vi "Tree_Get All Child Tags.vi"(8 "error in (no error)":errorcluster, 10 "Parent Tag":string, 11 "Tree Refnum":refnum<vi>) -> (0 "error out":errorcluster, 2 "All Child Tags":string[](array[string]), 3 "dup Tree Refnum":refnum<vi>)   [LabVIEW 2017]
doc: "This VI takes a tree reference and a parent tag value, and returns a string array with the tags of all children (including sub-children) of the given parent tag."
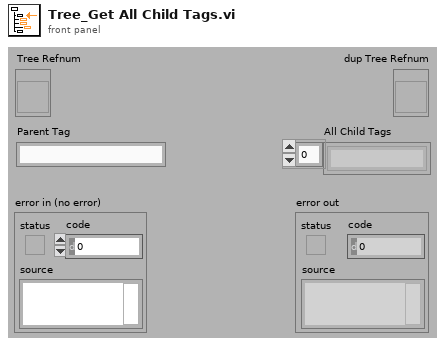
[diagram p1: front panel]
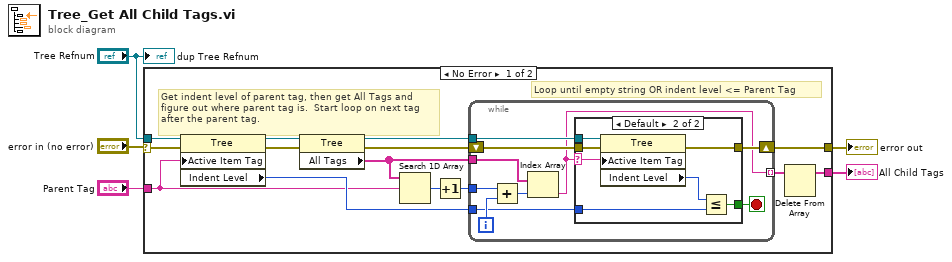
[diagram p0: block diagram]
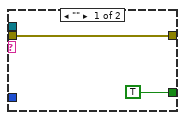
[diagram p2: hidden frame]
diagram:
  n1 = case shown="No Error" "error in (no error)" {
    selector: "error in (no error)" -> [w18 w39]
    tunnel: [w9 w39] -> w4
    tunnel: "Tree Refnum" -> [w19 _]
    tunnel: "Parent Tag" -> [w6 _]
    tunnel: [w11 _] -> w1
    frame No Error {
      # "Loop until empty string OR indent level <= Parent Tag"
      # "Get indent level of parent tag, then get All Tags and\nfigure out where parent tag is.  Start loop on next tag\nafter the parent tag."
      n2 = property class="Tree"(reference=w19, error in=w18, "Active Item Tag"=w6) -> (reference out=w16:refnum<vi>, error out=w17:errorcluster, "Indent Level"=w7:i32)
      n3 = property class="Tree"(reference=w16, error in=w17) -> (reference out=w8:refnum<vi>, error out=w10:errorcluster, "All Tags"=w14:string[])
      n4 = Search 1D Array(1D array=w14, element=w6) -> (index of element=w15:i32)  [unwired: 1 out]
      n5 = Increment(x=w15) -> (x+1=w13:i32)
      n6 = while {
        tunnel: w14 -> [w29]
        tunnel: w13 -> [w28]
        tunnel: [w20] -> w12 mode=indexing
        shift-right: [w23] -> w9
        shift-left: w10 -> [w25]
        tunnel: w8 -> [w24]
        tunnel: w7 -> [w22]
        i -> [w27]
        stop <- w21 stop-if-true
        n7 = Add(x=w28, y=w27) -> (x+y=w26:i32)
        n8 = Index Array(array=w29, index=w26) -> (element=w20:string)
        n9 = case shown="Default" w20 {
          selector: w20 -> [_ w32]
          tunnel: w25 -> [w31 w38]
          tunnel: w24 -> [_ w37]
          tunnel: [w31 w36] -> w23
          tunnel: w22 -> [_ w34]
          tunnel: [TRUE w33] -> w21
          frame "" {
          }
          frame Default {
            n10 = property class="Tree"(reference=w37, error in=w38, "Active Item Tag"=w32) -> (error out=w36:errorcluster, "Indent Level"=w35:i32)  [unwired: 1 out]
            n11 = Less Or Equal?(x=w35, y=w34) -> (x <= y?=w33:bool)
          }
        }
      }
      n12 = Delete From Array(array=w12) -> (array with subset deleted=w11:string[])  [unwired: 2 in, 1 out]
    }
    frame Error {
    }
  }
  "error out" <- w4
  "All Child Tags" <- w1
  "dup Tree Refnum" <- "Tree Refnum"
